vi "MARS_Update_FoM_Graph.vi"() -> (3 "FoM Graph":dbl[][](array[numeric]))   [LabVIEW 2015]
uses:
  Data_Analysis_subvis/MARS_Scan_Data_Analysis_global.vi
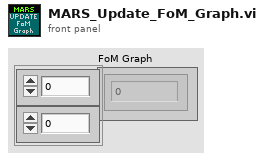
[diagram p1: front panel]
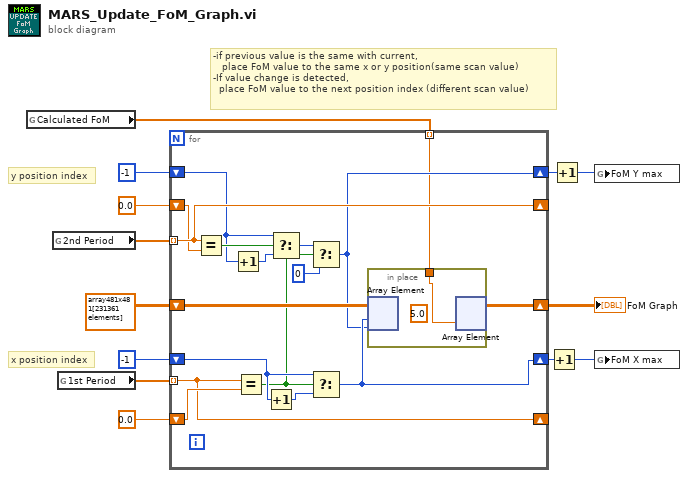
[diagram p0: block diagram]
diagram:
  # "x position index"
  # "y position index"
  # "-if previous value is the same with current, \n   place FoM value to the same x or y position(same scan value)\n-If value change is detected, \n  place FoM value to the next position index (different scan value)"
  n1 = global read "MARS_Scan_Data_Analysis_global.vi" "Calculated FoM"() -> (w1:dbl[])
  n2 = global read "MARS_Scan_Data_Analysis_global.vi" "2nd Period"() -> (w7:dbl[])
  n3 = global read "MARS_Scan_Data_Analysis_global.vi" "1st Period"() -> (w8:dbl[])
  n4 = for {
    tunnel: w7 -> [w30] mode=indexing
    shift-right: [w30] -> _
    shift-left: 0.0 ("Numeric Control") -> [w29]
    shift-right: [w26] -> w6
    shift-left: dbl[][] array481x481[231361 elements] ("1st period") -> [w27]
    tunnel: w8 -> [w24] mode=indexing
    shift-right: [w24] -> _
    shift-left: 0.0 ("Numeric Control") -> [w25]
    shift-right: [w19] -> w5
    shift-left: -1 ("Numeric Control") -> [w22]
    shift-right: [w16] -> w4
    shift-left: -1 ("Numeric Control") -> [w21]
    tunnel: w1 -> [w15] mode=indexing
    n5 = Equal?(x=w30, y=w29) -> (x = y?=w28:bool)
    n6 = Increment(x=w21) -> (x+1=w20:i32)
    n7 = Equal?(x=w24, y=w25) -> (x = y?=w14:bool)
    n8 = Increment(x=w22) -> (x+1=w23:i32)
    n9 = Select(t=w21, s=w28, f=w20) -> (s? t:f=w17:i32)
    n10 = Select(t=w17, s=w14, f=0) -> (s? t:f=w16:i32)
    n11 = Select(t=w22, s=w14, f=w23) -> (s? t:f=w19:i32)
    n12 = in-place {
      in-place-border: w15 -> [w31]
      (unwired) 5.0
      n13 = in-place-array #1(w27, w19, w16) -> ()  [unwired: 1 out]
      n14 = in-place-array #1(w31) -> (w26:dbl[][])  [unwired: 2 out]
    }
  }
  "FoM Graph" <- w6
  n15 = Increment(x=w5) -> (x+1=w2:i32)
  n16 = Increment(x=w4) -> (x+1=w3:i32)
  n17 = global write "MARS_Scan_Data_Analysis_global.vi" "FoM Y max"(w3) -> ()
  n18 = global write "MARS_Scan_Data_Analysis_global.vi" "FoM X max"(w2) -> ()
